vi "Instantiate.vi"(1 "vi ref":refnum<vi>) -> (0 "vi ref":refnum<vi>)   [LabVIEW 2022 SP3, in "Enclave.lvlib"]
uses:
  Enclave.lvlib
  ))Channel.vi
  Operation.ctl
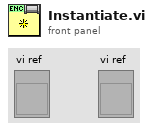
[diagram p1: front panel]
types:
  T1 = typedef "Enclave.lvlib/Operation.ctl" = enum16{"Get Core", "Init", "Close"}
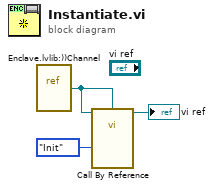
[diagram p0: block diagram]
diagram:
  n1 = vi-ref "Enclave.lvlib:))Channel.vi"() -> (w3:refnum<vi>)
  n2 = call-by-ref "?"(reference=w3, "This VI in"=w3, "Operation"=Operation."Init") -> (reference out=→"vi ref":refnum<vi>)  [unwired: 13 in, 3 out]
